vi "Loop Timing.vi"() -> ()   [LabVIEW 2019]
panel:
  in  "stop":bool
  out "Random Number":dbl
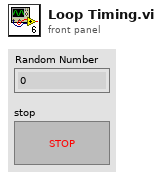
[diagram p1: front panel]
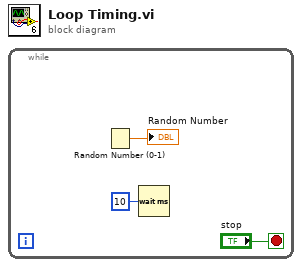
[diagram p0: block diagram]
diagram:
  n1 = while {
    stop <- "stop" stop-if-true
    n2 = Random Number (0-1)() -> (number: 0 to 1=→"Random Number":dbl)
    n3 = Wait (ms)(milliseconds to wait=u32 10) -> ()  [unwired: 1 out]
  }
